vi "allStringsFreq.vi"() -> (3 "array of frequencies":dbl[](array[numeric]))   [LabVIEW 2019]
panel:
  in  "Numeric":dbl
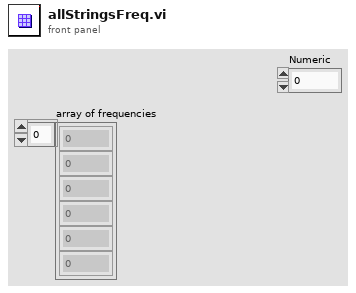
[diagram p1: front panel]
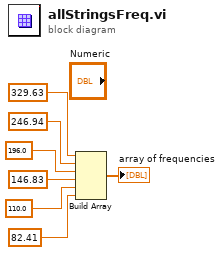
[diagram p0: block diagram]
diagram:
  n1 = Build Array(329.63 ("element"), 246.94 ("element"), 196.0 ("element"), 146.83 ("element"), 110.0 ("element"), 82.41 ("element")) -> (→"array of frequencies":dbl[])
